vi "autoDestroyFunction.vi"(11 "command in":string[](array[string])) -> ()   [LabVIEW 2013]
panel:
  out "element":string
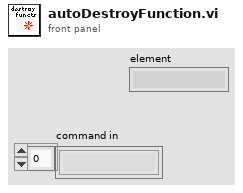
[diagram p1: front panel]
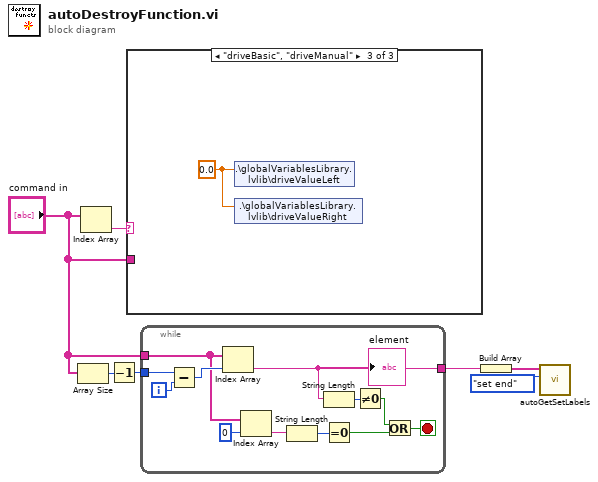
[diagram p0: block diagram]
diagram:
  n1 = Array Size(array="command in") -> (size(s)=w6:i32)
  n2 = Index Array(array="command in") -> (element=w7:string)  [unwired: 1 in]
  n3 = Decrement(x=w6) -> (x-1=w5:i32)
  n4 = case shown="\"driveBasic\", \"driveManual\"" w7 {
    tunnel: "command in" -> [_ _ _]
    frame "testFunct" {
    }
    frame Default {
    }
    frame "driveBasic", "driveManual" {
      w8 = 0.0 ("Output")
      n5 = shared-variable ".\\globalVariablesLibrary.lvlib\\driveValueLeft"(w8) -> ()  [unwired: 1 in, 1 out]
      n6 = shared-variable ".\\globalVariablesLibrary.lvlib\\driveValueRight"(w8) -> ()  [unwired: 1 in, 1 out]
    }
  }
  n7 = while {
    tunnel: "command in" -> [w15]
    tunnel: w5 -> [w19]
    tunnel: [w16] -> w2
    i -> [w20]
    stop <- w9 stop-if-true
    n8 = Subtract(x=w19, y=w20) -> (x-y=w18:i32)
    n9 = Index Array(array=w15, index=w18) -> (element=w16:string)
    "element" <- w16
    n10 = Index Array(array=w15, index=0) -> (element=w13:string)
    n11 = String Length(string=w13) -> (length=w12:i32)
    n12 = String Length(string=w16) -> (length=w17:i32)
    n13 = Equal To 0?(x=w12) -> (x = 0?=w11:bool)
    n14 = Not Equal To 0?(x=w17) -> (x != 0?=w10:bool)
    n15 = Or(x=w10, y=w11) -> (x .or. y?=w9:bool)
  }
  n16 = Build Array(w2) -> (w1:string[])
  n17 = call "autoGetSetLabels.vi"("option in"=enum16{"get", "set", "remove", "set end"}."set end", "label in"=w1) -> ()  [unwired: 9 in, 1 out]
